vi "SIAM-convertReturnToReadable.vi"(8 "error in (no error)":errorcluster, 11 "Return":u32[](array[numeric]) format="%.0x") -> (0 "error out":errorcluster, 3 "Readable":string)   [LabVIEW 2011]
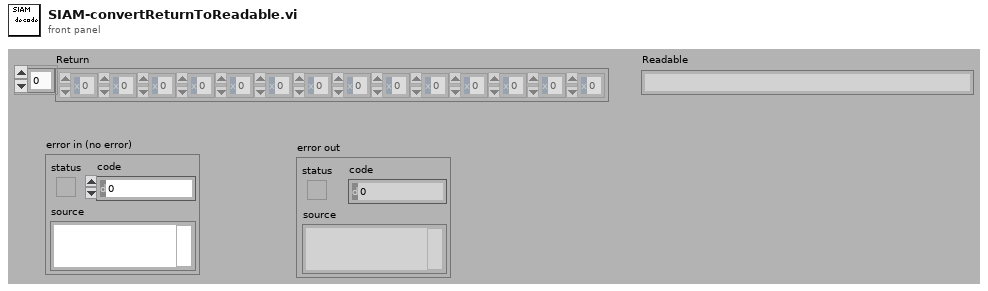
[diagram p1: front panel]
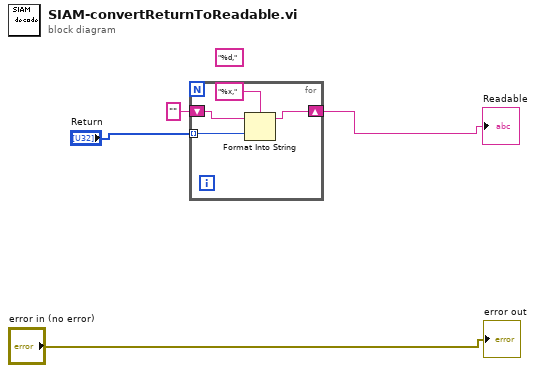
[diagram p0: block diagram]
diagram:
  (unwired) "%d," ("format string")
  n1 = for {
    tunnel: "Return" -> [w8] mode=indexing
    shift-right: [w5] -> w4
    shift-left: "" -> [w6]
    n2 = Format Into String(format string="%x,", initial string=w6, w8) -> (resulting string=w5:string)  [unwired: 1 in, 1 out]
  }
  "Readable" <- w4
  "error out" <- "error in (no error)"
